vi "SigmoidArr.vi"(1 "x":dbl[][](array[numeric])) -> (0 "Sigmoid":dbl[][](array[numeric]))   [LabVIEW 2021]
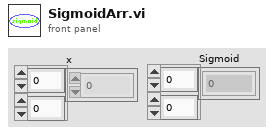
[diagram p1: front panel]
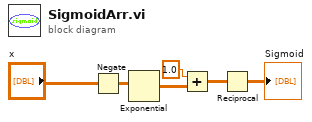
[diagram p0: block diagram]
diagram:
  n1 = Negate(x="x") -> (-x=w6:dbl[][])
  n2 = Exponential(1:w6) -> (0:w4:dbl[][])
  n3 = Add(x=1.0, y=w4) -> (x+y=w3:dbl[][])
  n4 = Reciprocal(x=w3) -> (1/x=→"Sigmoid":dbl[][])
